vi "CurrentSenseController.vi"() -> ()   [LabVIEW 2012]
uses:
  <instrlib>/niScope/Controls/niScope vertical coupling.ctl
  <instrlib>/niScope/Controls/niScope trigger source.ctl
  <vilib>/Instr/_visa.llb/VISA Configure Serial Port (Instr).vi
  <instrlib>/niScope/Acquire/niScope Multi Read Cluster.vi
  <vilib>/Utility/file.llb/Write To Spreadsheet File (DBL).vi
panel:
  in  "Tab Control":enum32{"View", "Configuration"}(tab)
  in  "Log Data":bool
  out "Resistor Confirm":bool
  in  "Boolean":bool=TRUE
  in  "Control-only":bool
  in  "Analog Triggering":bool
  in  "Trigger Slope":u32(ring) items=["Positive", "Negative"]
  out "Current Draw (CH 0)":cluster{i32, "xIncrement":dbl, dbl[][]}(graph)
  in  "Length of Capture (s)":dbl(slide)=0.01 scale=1e-06..1.0
  in  "Trigger Position (% of plot)":dbl(slide)=25.0 scale=0.0..100.0
  in  "Level (mA)":dbl(slide) step=0.1 scale=0.0..500.0
  in  "Sense Resistor":u32(ring)=1 items=["Auto", "500mA", "200mA", "100mA", "50mA", "10mA", "1mA"]
  in  "Set":bool
  in  "stop":bool
  in  "Triggering":bool
  in  "Minimum Y":dbl(slide) step=0.01 scale=0.0..500.0
  out "Mean (mA)":dbl format="%0.2f"
  out "STD Deviation":dbl format="%0.2f"
  in  "trigger source":T1="1" caption="Trigger Source"
  out "Triggering Pin (CH 1)":cluster{ext, "xIncrement":dbl, "wfm":dbl[]}(graph)
  in  "Trigger Type":i32(ring)=2 items=["Risky Trigger"=1, "Auto Trigger"=2]
  in  "Timeout":dbl=5.0
  in  "vertical coupling":T2=1 caption="Vertical Coupling" items=["AC", "DC"]
  in  "IVI Logical Name":refnum<k15>="PXI1Slot7"
  in  "flow control":u16(ring) items=["None"=0, "XON/XOFF"=1, "RTS/CTS"=2, "DTR/DSR"=4]
  in  "stop bits":u16(ring)=10 items=["1.0"=10, "1.5"=15, "2.0"=20]
  in  "parity":u16(ring) items=["None", "Odd", "Even", "Mark", "Space"]
  in  "data bits":u16=8 min=5 max=8 step=1
  in  "baud rate":u32=115200
  in  "Serial Port":refnum<visa-resource-name>="COM3"
  out "error out 2":errorcluster caption="serial error" {"code" format="%.0x"}
  in  "Probe Impedance":enum8{"1M", "50ohm"}(ring)
  in  "Vertical Range (V)":dbl(slide)=4.0 scale=1.0..10.0
  out "error out":errorcluster caption="oscilloscope error" {"code" format="%.0x"}
  # "Serial Settings"
  # "Oscilloscope Controls"
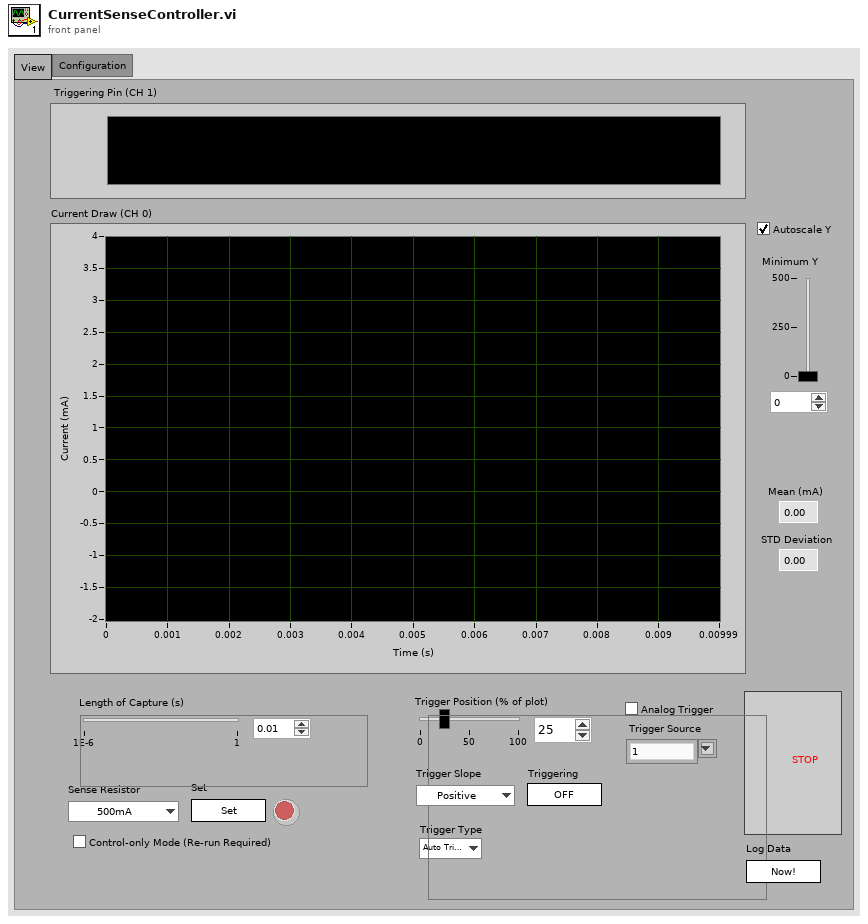
[diagram p1: front panel]
types:
  T1 = typedef "niScope trigger source.ctl" = string
  T2 = typedef "niScope vertical coupling.ctl" = i32
  T3 = enum8{"Enabled", "Disabled", "Disabled and Grayed Out"}
  T4 = cluster{"relativeInitialX":dbl, "xIncrement":dbl, "wfm":dbl[]}[]
  T5 = cluster{"relativeInitialX":dbl, "xIncrement":dbl, "wfm":dbl[]}
  T6 = cluster{"Numeric":i32, "xIncrement":dbl, "Array":dbl[]}
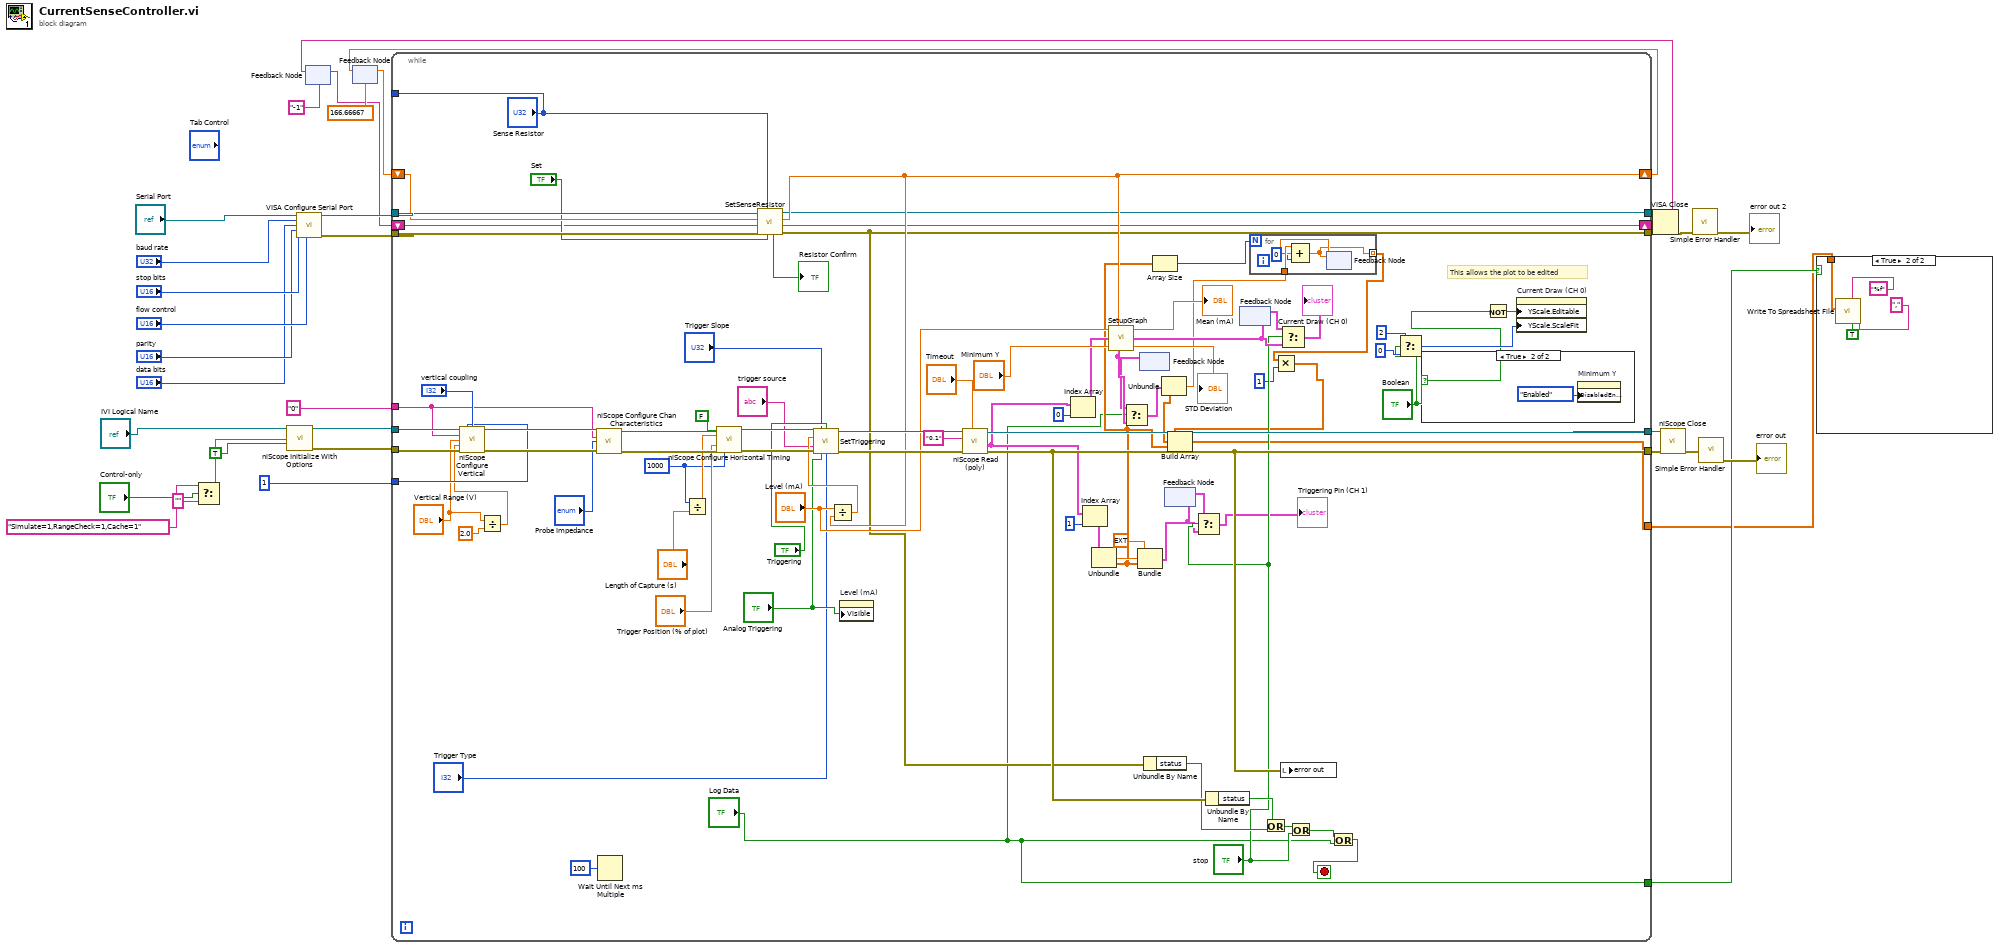
[diagram p0: block diagram]
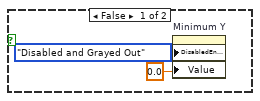
[diagram p3: hidden frame]
diagram:
  n1 = Select(t="Simulate=1,RangeCheck=1,Cache=1" ("option string"), s="Control-only", f="") -> (s? t:f=w11:string)
  n2 = call <instrlib>:"niScope Initialize With Options.vi"("resource name"="IVI Logical Name", "option string"=w11, "reset device"=TRUE) -> ("instrument handle"=w16:refnum<k15>, "error out"=w15:errorcluster)  [unwired: 11 in]
  n3 = call-poly "VISA Configure Serial Port"("VISA resource name"="Serial Port", "baud rate (9600)"="baud rate", "data bits (8)"="data bits", "parity (0:none)"="parity", "stop bits (10: 1 bit)"="stop bits", "flow control (0:none)"="flow control") -> ("VISA resource name out"=w28:refnum<visa-resource-name>, "error out"=w27:errorcluster)  [unwired: 8 in]
  n4 = feedback #1("-1" ("Current Channel")) -> (w6:string)
  n5 = feedback #2(166.66667 ("CurrentScalingFactor")) -> (w18:dbl)
  n6 = while {
    tunnel: w28 -> [w93]
    tunnel: w27 -> [w92]
    tunnel: w16 -> [w118]
    tunnel: w15 -> [w116]
    tunnel: "0" -> [w102]
    tunnel: [w110] -> w25
    tunnel: [w101] -> w24
    tunnel: 1 -> [w108]
    shift-right: [w88] -> w19
    shift-left: w18 -> [w91]
    tunnel: ["Sense Resistor"] -> _
    tunnel: [w65] -> w8
    tunnel: [w64] -> w7
    shift-right: [w61] -> w5
    shift-left: w6 -> [w62]
    tunnel: [w36] -> w1
    tunnel: ["Log Data"] -> w2
    stop <- w37 stop-if-true
    w94 = 1000
    # "This allows the plot to be edited"
    n7 = Divide(x="Vertical Range (V)", y=2.0) -> (x/y=w52:dbl)
    n8 = call <instrlib>:"niScope Configure Vertical.vi"("instrument handle"=w118, "probe attenuation"=w108, "vertical coupling"="vertical coupling", "channels"=w102, "vertical range"="Vertical Range (V)", "vertical offset"=w52, "error in"=w116) -> ("instrument handle out"=w117:refnum<k15>, "error out"=w115:errorcluster)  [unwired: 7 in]
    n9 = call <instrlib>:"niScope Configure Chan Characteristics.vi"("instrument handle"=w117, "channels"=w102, "input impedance"="Probe Impedance", "error in"=w115) -> ("instrument handle out"=w114:refnum<k15>, "error out"=w113:errorcluster)  [unwired: 10 in]
    n10 = Wait Until Next ms Multiple(millisecond multiple=u32 100) -> ()  [unwired: 1 out]
    n11 = Divide(x=w94, y="Length of Capture (s)") -> (x/y=w96:dbl)
    n12 = call <instrlib>:"niScope Configure Horizontal Timing.vi"("instrument handle"=w114, "enforce realtime"=FALSE, "min sample rate"=w96, "reference position"="Trigger Position (% of plot)", "error in"=w113, "min record length"=w94) -> ("instrument handle out"=w104:refnum<k15>, "error out"=w106:errorcluster)  [unwired: 8 in]
    n13 = call "SetSenseResistor.vi"("Set Button"="Set", "Sense Resistor"="Sense Resistor", "error in"=w92, "Previous Channel"=w62, "PastScalingFactor"=w91, "VISA resource name"=w93) -> ("error out 2"=w64:errorcluster, "Current Channel"=w61:string, "CurrentScalingFactor"=w88:dbl, "VISA resource name out"=w65:refnum<visa-resource-name>, "isCorrect"=→"Resistor Confirm":bool)  [unwired: 1 in]
    n14 = Divide(x="Level (mA)", y=w88) -> (x/y=w90:dbl)
    n15 = call "SetTriggering.vi"("instrument handle out"=w104, "trigger slope"="Trigger Slope", "Triggering?"="Triggering", "Trigger Level"=w90, "trigger source"="trigger source", "error in"=w106, "Analog Triggering"="Analog Triggering", "Triggering:Trigger Modifier"="Trigger Type") -> ("instrument handle out 2"=w103:refnum<k15>, "error out"=w105:errorcluster)  [unwired: 6 in]
    n16 = property on="Level (mA)" class="Slide (strict)"("Visible"="Analog Triggering") -> ()  [unwired: 2 in, 2 out]
    n17 = call-poly <instrlib>:"niScope Read (poly).vi"("timeout"="Timeout", "error in"=w105, "channels"="0,1", "instrument handle"=w103) -> ("error out"=w101:errorcluster, "waveform"=w81:T4, "instrument handle out"=w110:refnum<k15>)  [unwired: 4 in, 1 out]
    n18 = Index Array(array=w81, index=0) -> (element=w83:T5)
    n19 = Index Array(array=w81, index=1) -> (element=w58:T5)
    n20 = Unbundle(w58) -> ("xIncrement"=w57:dbl, "wfm"=w43:dbl[])  [unwired: 1 out]
    n21 = call "SetupGraph.vi"("trigger level"="Level (mA)", "Scaling Factor"=w88, "input capture cluster"=w83, "Minimum Y"="Minimum Y") -> ("current only plot"=w48:T6, "mean"=→"Mean (mA)":dbl, "output plot"=w75:cluster{i32, "xIncrement":dbl, dbl[][]}, "standard deviation"=→"STD Deviation":dbl)  [unwired: 1 in, 1 out]
    n22 = Bundle(ext 0.0, "xIncrement"=w57, "wfm"=w43) -> (w55:cluster{ext, "xIncrement":dbl, "wfm":dbl[]})  [unwired: 1 in]
    n23 = feedback #3() -> (w47:T6)  [unwired: 1 in]
    n24 = Select(t=w47, s="Log Data", f=w48) -> (s? t:f=w46:T6)
    n25 = feedback-in #3(w48) -> ()
    n26 = Unbundle By Name(w64) -> ("status"=w99:bool)
    n27 = Array Size(array=w43) -> (size(s)=w42:i32)
    n28 = Unbundle(w46) -> ("xIncrement"=w41:dbl, "Array"=w45:dbl[])  [unwired: 1 out]
    n29 = feedback #4() -> (w73:cluster{ext, "xIncrement":dbl, "wfm":dbl[]})  [unwired: 1 in]
    n30 = feedback-in #4(w55) -> ()
    n31 = Select(t=w73, s="stop", f=w55) -> (s? t:f=→"Triggering Pin (CH 1)":cluster{ext, "xIncrement":dbl, "wfm":dbl[]})
    n32 = Unbundle By Name(w101) -> ("status"=w98:bool)
    n33 = feedback #5() -> (w74:cluster{i32, "xIncrement":dbl, dbl[][]})  [unwired: 1 in]
    n34 = feedback-in #5(w75) -> ()
    n35 = for {
      N: w42 -> [_]
      tunnel: w41 -> [w122]
      tunnel: [w119] -> w40 mode=indexing
      n36 = feedback #6() -> (w121:dbl)  [unwired: 1 in]
      n37 = Compound Arithmetic op=ADD(w122, w121, 0) -> (w119:dbl)
      n38 = feedback-in #6(w119) -> ()
    }
    n39 = Or(x=w98, y=w99) -> (x .or. y?=w107:bool)
    n40 = Multiply(x=w40, y=1) -> (x*y=w39:dbl[])
    n41 = Build Array(w39, w45, w43) -> (w36:dbl[][])
    n42 = Select(t=w74, s="stop", f=w75) -> (s? t:f=→"Current Draw (CH 0)":cluster{i32, "xIncrement":dbl, dbl[][]})
    n43 = local write "error out"(w101) -> ()
    n44 = Or(x=w107, y="stop") -> (x .or. y?=w38:bool)
    n45 = Or(x=w38, y="Log Data") -> (x .or. y?=w37:bool)
    n46 = Select(t=u8 2, s="Boolean", f=u8 0) -> (s? t:f=w69:u8)
    n47 = case shown="True" "Boolean" {
      frame False {
        n48 = property on="Minimum Y" class="Slide (strict)"("DisabledEnum"=T3."Disabled and Grayed Out" ("Disabled"), "Value"=0.0 ("Minimum Y")) -> ()  [unwired: 2 in, 2 out]
      }
      frame True {
        n49 = property on="Minimum Y" class="Slide (strict)"("DisabledEnum"=T3."Enabled" ("Disabled")) -> ()  [unwired: 2 in, 2 out]
      }
    }
    n50 = Not(x="Boolean") -> (.not. x?=w68:bool)
    n51 = property on="Current Draw (CH 0)" class="WFGraph (strict)"("YScale.Editable"=w68, "YScale.ScaleFit"=w69) -> ()  [unwired: 2 in, 2 out]
  }
  n52 = feedback-in #1(w5) -> ()
  n53 = feedback-in #2(w19) -> ()
  n54 = VISA Close(VISA resource name=w8, error in (no error)=w7) -> (error out=w22:errorcluster)
  n55 = call <instrlib>:"niScope Close.vi"("instrument handle"=w25, "error in"=w24) -> ("error out"=w3:errorcluster)  [unwired: 13 in]
  n56 = call <vilib>:"Simple Error Handler.vi"("error in (no error)"=w22) -> ("error out"=→"error out 2":errorcluster)  [unwired: 4 in, 4 out]
  n57 = call <vilib>:"Simple Error Handler.vi"("error in (no error)"=w3) -> ("error out"=→"error out":errorcluster)  [unwired: 4 in, 4 out]
  n58 = case shown="True" w2 {
    tunnel: w1 -> [_ w126]
    frame False {
    }
    frame True {
      n59 = call-poly <vilib>:"Write To Spreadsheet File.vi"("delimiter (\\t)"=",", "transpose? (no:F)"=TRUE, "format (%.3f)"="%f", "2D data"=w126) -> ()  [unwired: 4 in, 1 out]
    }
  }
